vi "Metrolab_main_SF_and_dipoles.vi"() -> ()   [LabVIEW 2017]
panel:
  out "Labels":string[](array[string])=["I_D1 (A)", "I_D2(A)", "I_SFDC (A)", "I_RF (A)", "l (mm)", "z (mm)", "Bx (mT)", "By (mT)", "Bz (mT)", "|B| (mT)"]
  in  "I_D2 (A)":dbl=112.0
  in  "I_D1 (A)":dbl=112.0
  out "Graph (Bx)":cluster{timestamp[], dbl[]}(graph)={[timestamp(3708568369.45642 s since 1904-01-01), timestamp(3708568377.924761 s since 1904-01-01)], [-0.02, -0.01]} caption="XY Graph"
  out "XY Graph":cluster{dbl[], dbl[]}(graph)
  in  "I_RF (A)":dbl=112.0
  in  "I_SFDC (A)":dbl=112.0
  out "Cycle #":i32
  in  "COMMENT":string="THM7025_zscan_practice"
  out "Graph (Bz)":cluster{timestamp[], dbl[]}(graph)={[timestamp(3708568369.45642 s since 1904-01-01), timestamp(3708568377.924761 s since 1904-01-01)], [0.25, 0.24]} caption="XY Graph"
  out "Graph (By)":cluster{timestamp[], dbl[]}(graph)={[timestamp(3708568369.45642 s since 1904-01-01), timestamp(3708568377.924761 s since 1904-01-01)], [-0.01, -0.01]} caption="XY Graph"
  in  "Stop":bool=TRUE
  out "Graph (z)":cluster{timestamp[], dbl[]}(graph)={[timestamp(3708568369.45642 s since 1904-01-01), timestamp(3708568377.924761 s since 1904-01-01)], [-0.02, -0.01]} caption="XY Graph"
  out "Z (mm) = 600 - L":dbl=378.0 format="%_5f"
  in  "L (mm)":dbl=112.0
  in  "Measure":bool
  out "File Error Out":errorcluster
  in  "base path":path=path "C:/LabVIEW/DATA/J-PARC_202203"
  in  "error in (no error)":errorcluster caption="エラー入力（エラーなし）"
  out "error out":errorcluster caption="エラー出力" {"code" format="%.0x"}
  in  "VISA resource name":refnum<visa-resource-name>="COM4"
  out "Results":dbl[](array[numeric])=[-0.24, -0.01, -0.01, 0.24]
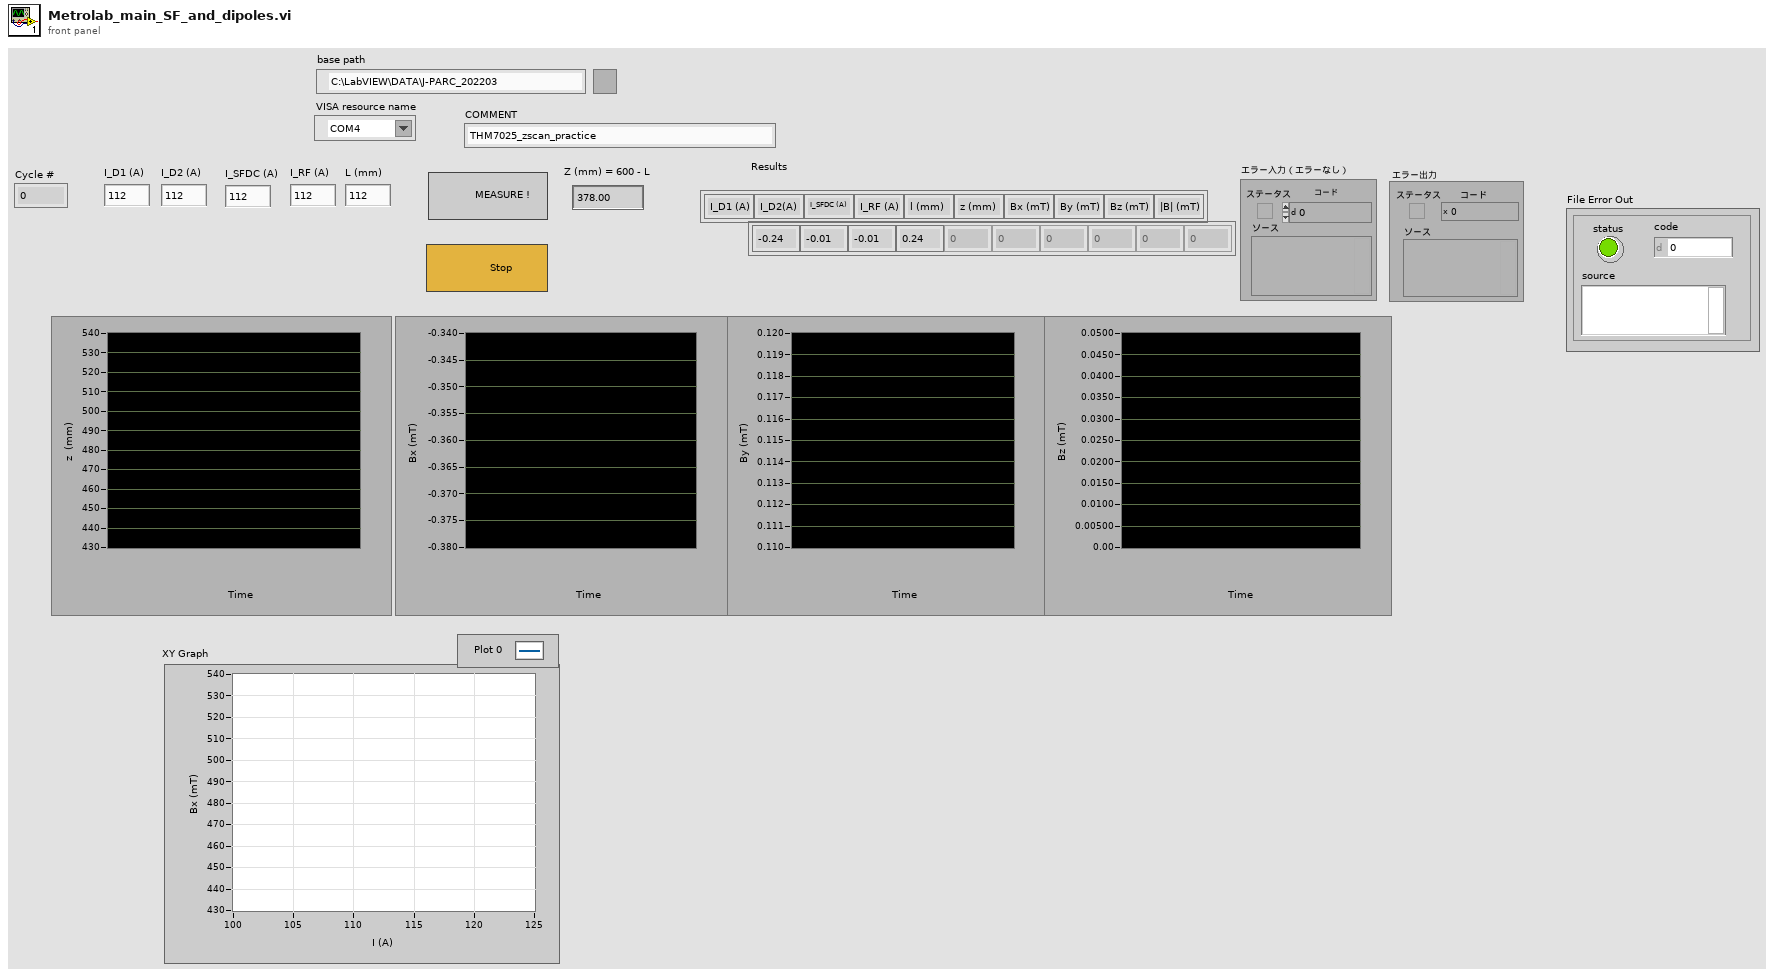
[diagram p1: front panel]
types:
  T1 = enum16{"open", "replace", "create", "open or create", "replace or create", "replace or create with confirmation"}
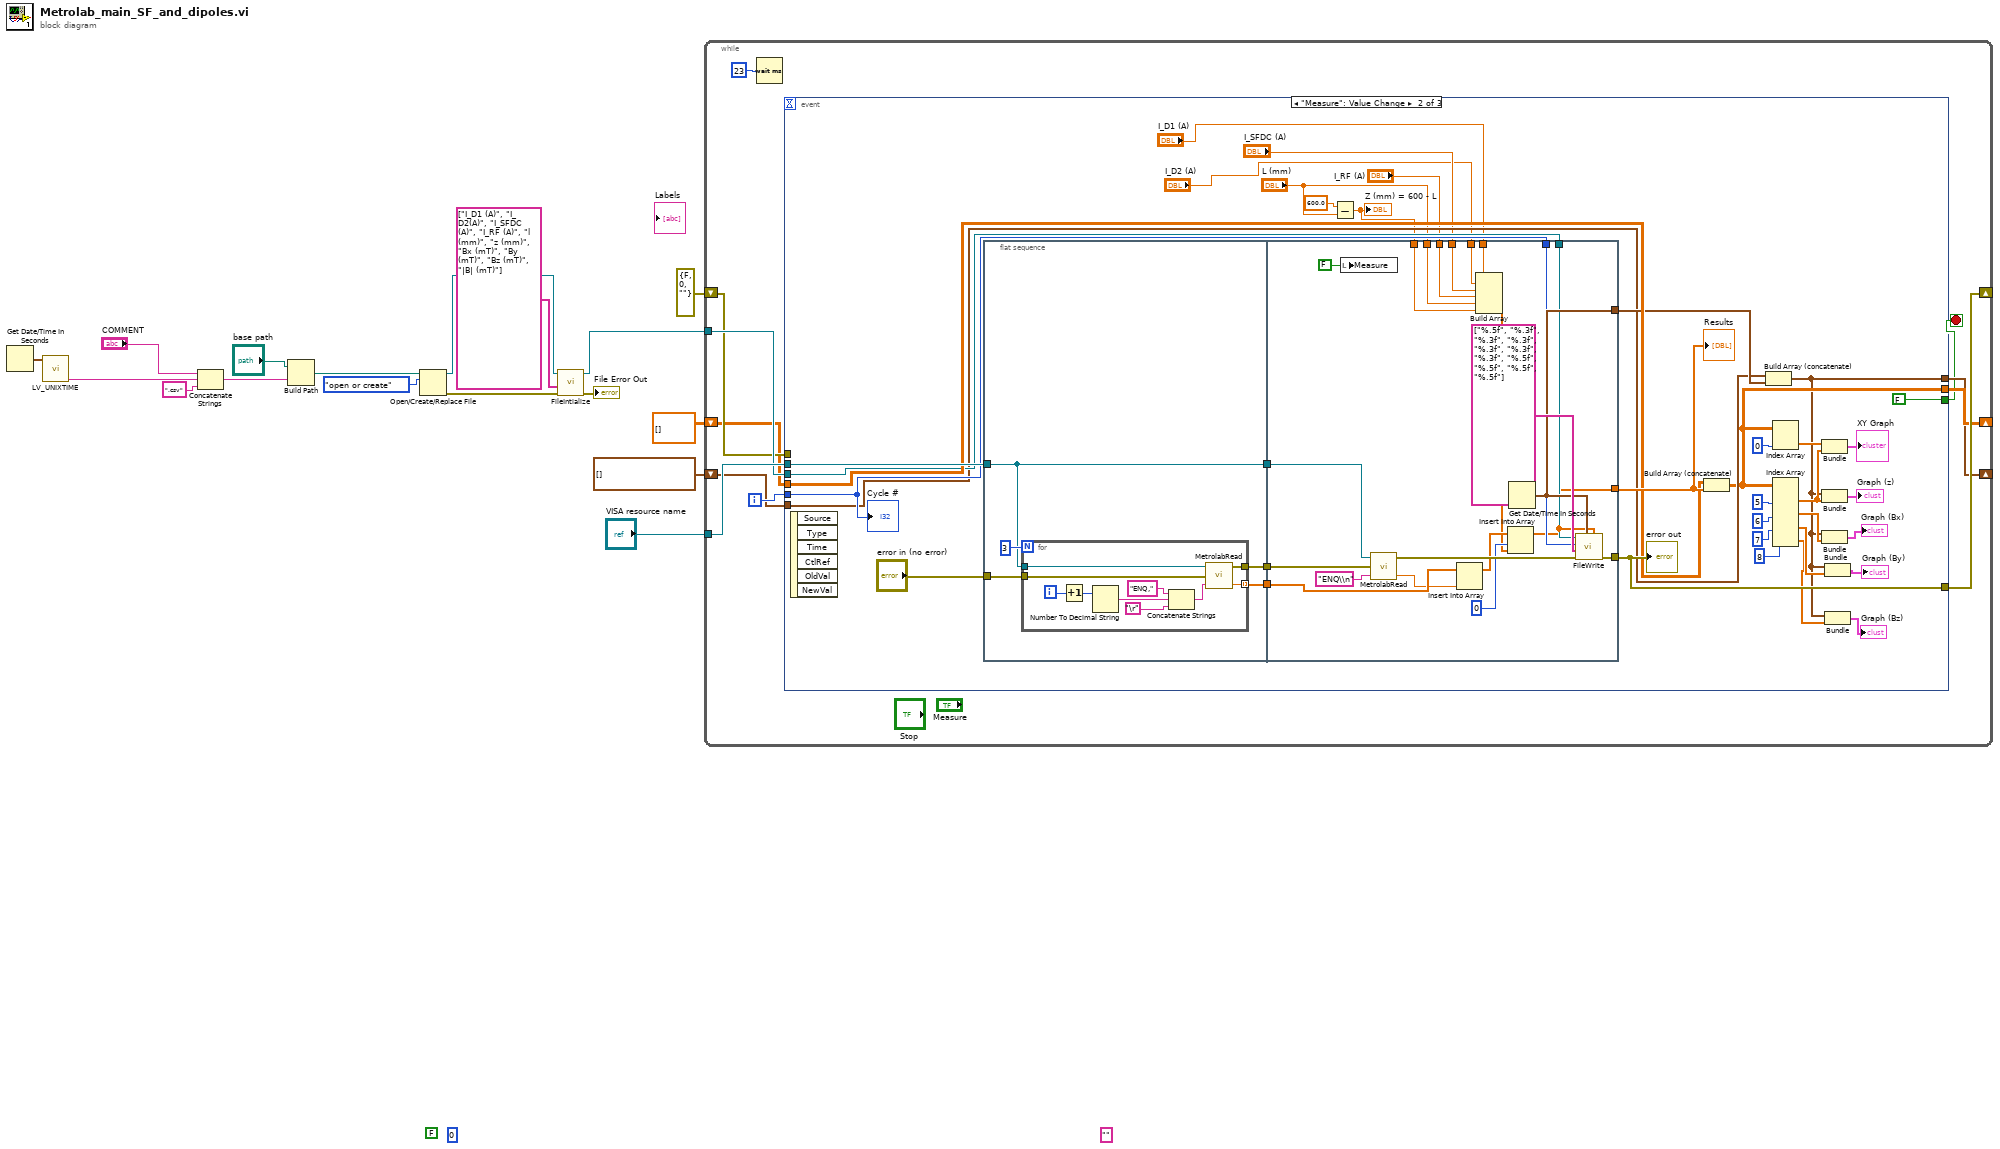
[diagram p0: block diagram]
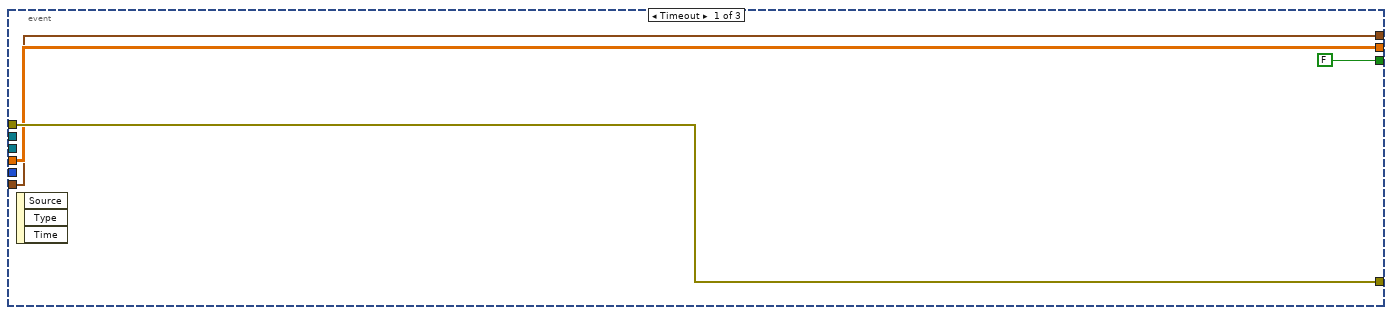
[diagram p2: hidden frame]
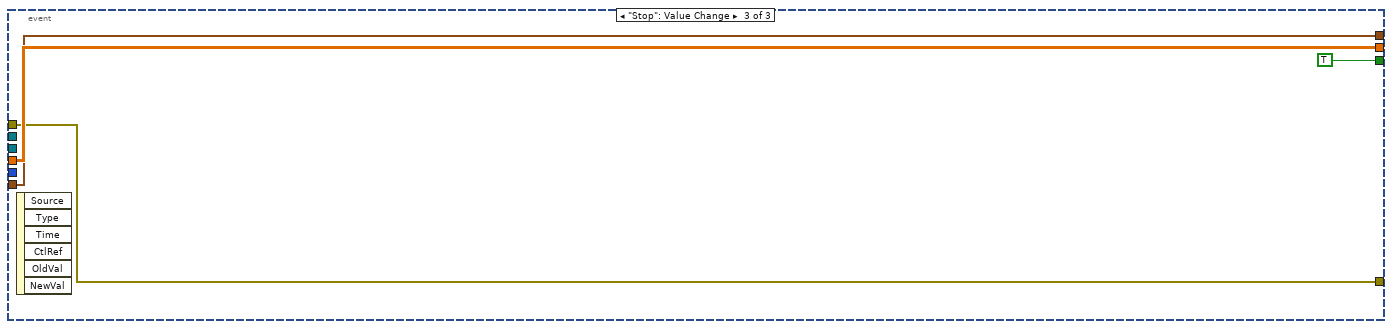
[diagram p3: hidden frame]
diagram:
  (unwired) FALSE ("status")
  (unwired) 0 ("code")
  (unwired) "" ("source")
  n1 = Get Date/Time In Seconds() -> (seconds since 1Jan1904=w14:timestamp)
  n2 = call "LV_UNIXTIME.vi"("current time"=w14) -> ("date/time string"=w11:string)  [unwired: 9 in, 1 out]
  n3 = Concatenate Strings("COMMENT", w11, ".csv" ("string")) -> (w9:string)
  n4 = Build Path(base path="base path", name or relative path=w9) -> (appended path=w13:path)
  n5 = Open/Create/Replace File(file path (use dialog)=w13, operation (0:open)=T1."open or create") -> (refnum out=w6:refnum<file>, error out=w7:errorcluster)  [unwired: 4 in, 1 out]
  n6 = call "FileIntialize.vi"("Error In"=w7, "Labels"=string[] ["I_D1 (A)", "I_D2(A)", "I_SFDC (A)", "I_RF (A)", "l (mm)", "z (mm)", "Bx (mT)", "By (mT)", "Bz (mT)", "|B| (mT)"], "refnum in"=w6) -> ("Error Out"=→"File Error Out":errorcluster, "File Refnum"=w4:refnum<file>)  [unwired: 7 in]
  n7 = while {
    tunnel: "VISA resource name" -> [w27]
    tunnel: w4 -> [w26]
    shift-right: [w24] -> _
    shift-left: errorcluster {"status"=FALSE, "code"=0, "source"=""} ("Error Out") -> [w23]
    shift-right: [w21] -> _
    shift-left: dbl[][] [] -> [w22]
    shift-right: [w20] -> _
    shift-left: timestamp[] [] -> [w19]
    i -> [w25]
    stop <- w18 stop-if-true
    n8 = Wait (ms)(milliseconds to wait=u32 23) -> ()  [unwired: 1 out]
    n9 = event shown="[1] \"Measure\": Value Change" {
      selector: _ -> [_ _ _]
      dyn-events: _ -> [_ _ _]
      timeout: _ -> [_ _ _]
      tunnel: w27 -> [_ w65 _]
      tunnel: w26 -> [_ w56 _]
      tunnel: w25 -> [_ w55 _]
      tunnel: [w32 w63 w107] -> w24
      tunnel: w23 -> [w32 _ w107]
      tunnel: w22 -> [w31 w61 w109]
      tunnel: [w31 w45 w109] -> w21
      tunnel: [w29 w35 w108] -> w20
      tunnel: w19 -> [w29 w54 w108]
      tunnel: [FALSE ("Stop") FALSE ("Stop") TRUE ("Stop")] -> w18
      event Timeout {
        n10 = event-data() -> ()  [unwired: 1 in, 3 out]
      }
      event "Measure": Value Change {
        n11 = event-data() -> ()  [unwired: 1 in, 6 out]
        n12 = flat-sequence {
          tunnel: [w70] -> w69
          tunnel: [w73] -> w68
          tunnel: [w72] -> w67
          tunnel: "error in (no error)" -> [w71]
          tunnel: w65 -> [w70]
          tunnel: w69 -> [w106]
          tunnel: w68 -> [w105]
          tunnel: w67 -> [w103]
          tunnel: [w87] -> w62
          tunnel: [w99] -> w63
          tunnel: [w98] -> w57
          tunnel: w56 -> [w97]
          tunnel: w55 -> [w96]
          tunnel: "L (mm)" -> [w95]
          tunnel: w51 -> [w94]
          tunnel: "I_SFDC (A)" -> [w90]
          tunnel: "I_RF (A)" -> [w89]
          tunnel: "I_D1 (A)" -> [w86]
          tunnel: "I_D2 (A)" -> [w85]
          frame #0 {
            n13 = for {
              N: 3 -> [_]
              tunnel: w70 -> [w84]
              tunnel: [w80] -> w72 mode=indexing
              tunnel: [w76] -> w73
              tunnel: w71 -> [w75]
              i -> [w77]
              n14 = Increment(x=w77) -> (x+1=w78:i32)
              n15 = Number To Decimal String(number=w78) -> (decimal integer string=w81:string)  [unwired: 1 in]
              n16 = Concatenate Strings("ENQ,", w81, "\r") -> (w82:string)
              n17 = call "MetrolabRead.vi"("Input string"=w82, "error in (no error)"=w75, "VISA resource name"=w84) -> ("B value [mT]"=w80:dbl, "error out"=w76:errorcluster)  [unwired: 1 out]
            }
          }
          frame #1 {
            n18 = local write "Measure"(FALSE ("Value (Signaling)")) -> ()
            n19 = call "MetrolabRead.vi"("Input string"="ENQ\\n", "error in (no error)"=w105, "VISA resource name"=w106) -> ("B value [mT]"=w102:dbl, "error out"=w100:errorcluster)  [unwired: 1 out]
            n20 = Insert Into Array(array=w103, new element=w102) -> (w91:dbl[])  [unwired: 1 in]
            n21 = Build Array(w86, w85, w90, w89, w95, w94) -> (w88:dbl[])
            n22 = Insert Into Array(array=w91, index=0, new element=w88) -> (w87:dbl[])
            n23 = Get Date/Time In Seconds() -> (seconds since 1Jan1904=w98:timestamp)
            n24 = call "FileWrite.vi"("DataArray"=w87, "Time Stamp"=w98, "Error In"=w100, "FileFormat"=string[] ["%.5f", "%.3f", "%.3f", "%.3f", "%.3f", "%.3f", "%.3f", "%.5f", "%.5f", "%.5f", "%.5f"], "Index"=w96, "refnum in"=w97) -> ("Error Out"=w99:errorcluster)  [unwired: 4 in, 1 out]
          }
        }
        n25 = Subtract(x=600.0, y="L (mm)") -> (x-y=w51:dbl)
        "Z (mm) = 600 - L" <- w51
        n26 = Build Array (concatenate)(w61, w62) -> (w45:dbl[][])
        n27 = Build Array (concatenate)(w54, w57) -> (w35:timestamp[])
        n28 = Index Array(array=w45, index (col)=0 ("disabled index (col)")) -> (element=w43:dbl[])  [unwired: 1 in]
        n29 = Index Array(array=w45, index (col) #1=5 ("disabled index (col)"), index (col) #2=6 ("disabled index (col)"), index (col) #3=7 ("disabled index (col)"), index (col) #4=8 ("index (col)")) -> (element #1=w42:dbl[], element #2=w49:dbl[], element #3=w48:dbl[], element #4=w39:dbl[])  [unwired: 4 in]
        n30 = Bundle(w43, w42) -> (→"XY Graph":cluster{dbl[], dbl[]})  [unwired: 1 in]
        n31 = Bundle(w35, w42) -> (→"Graph (z)":cluster{timestamp[], dbl[]})  [unwired: 1 in]
        n32 = Bundle(w35, w49) -> (→"Graph (Bx)":cluster{timestamp[], dbl[]})  [unwired: 1 in]
        n33 = Bundle(w35, w48) -> (→"Graph (By)":cluster{timestamp[], dbl[]})  [unwired: 1 in]
        n34 = Bundle(w35, w39) -> (→"Graph (Bz)":cluster{timestamp[], dbl[]})  [unwired: 1 in]
        "Results" <- w62
        "error out" <- w63
        "Cycle #" <- w55
      }
      event "Stop": Value Change {
        n35 = event-data() -> ()  [unwired: 1 in, 6 out]
      }
    }
  }
